vi "Add Injector.vi"(7 "Max Shots":T1(ring)=enum."1", 8 "error in (no error)":errorcluster, 9 "Stages":string[](array[string])=["Boost", "Battery", "Off"], 10 "Controls":T3[](array[typedef]) {"Data Type" format="%.0x"}, 11 "Item Ref":T2=18446744073709551615 format="%.0x") -> (0 "error out":errorcluster, 3 "Item Ref out":T2=18446744073709551615 format="%.0x")   [LabVIEW 2019, in "Fuel Injector Analysis Addon System Explorer.lvlib"]
uses:
  Fuel Injector Analysis Addon System Explorer.lvlib
  <vilib>/NI VeriStand/Custom Device API/Custom Device Item Ref.ctl
  Addon Shared/Types/Register.Info.ctl
  Addon Shared/Types/FPGA Data Types.ctl
  Support Libraries/Injection Capture IP/Types/Injection.Global.Settings.ctl
  Addon Shared/Constants.vi
  <vilib>/NI VeriStand/Custom Device API/Set Item Property (Variant).vi
  <vilib>/NI VeriStand/Custom Device Tools/Custom Device Utility Library/NI VeriStand - Search for Item by GUID.vi
  <vilib>/NI VeriStand/Custom Device Tools/Custom Device Utility Library/NI VeriStand - Search for All Items by GUID.vi
  Addon Shared/Fuel Injector Analysis Addon Shared.lvlib
  <vilib>/NI VeriStand/Custom Device API/Custom Device API.lvlib
  <vilib>/NI VeriStand/Custom Device Tools/Custom Device Utility Library/Custom Device Utility Library.lvlib
panel:
  in  "Tags":string
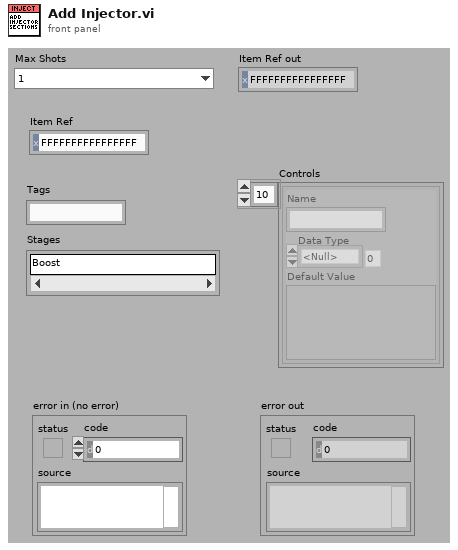
[diagram p1: front panel]
types:
  T1 = enum16{"0", "1", "2", "3", "4", "5", "6", "7", "8"}
  T2 = typedef "Custom Device API.lvlib/Custom Device Item Ref.ctl" = u64
  T3 = typedef "Fuel Injector Analysis Addon Shared.lvlib/Register.Info.ctl" = cluster{"Name":string, "Data Type":T4, "Default Value":variant}
  T4 = typedef "Fuel Injector Analysis Addon Shared.lvlib/FPGA Data Types.ctl" = enum8{"<Null>", "Injector.Core.Setting", "Injector.Global.Setting", "Injector.Mux.Setting", "Injector.Timing"}
  T5 = typedef "Injection.Global.Settings.ctl" = cluster{"Enable?":bool, "Initial Voltage Threshold":fxp<+/-,32,8>, "Event Dwell Limit":u16, "Voltage Gain":fxp<+/-,32,8>, "Current Gain":fxp<+/-,32,8>, "Filter Samples":u8, "Pretrigger Samples":u8, "Active Edge":bool}
  T6 = cluster{"Voltage Offset":fxp<+/-,32,8>, "Current Offset":fxp<+/-,32,8>}
  T7 = typedef "Custom Device API.lvlib/Custom Device Item Info.ctl" = cluster{"Name":string, "Is Channel":bool, "GUID":string, "Is Waveform":bool}
  T8 = typedef "Fuel Injector Analysis Addon Shared.lvlib/Main Settings.ctl" = cluster{"RIO Device Address":string, "Local bitfile path":path, "RT bitfile path":path, "Number of injectors":u16}
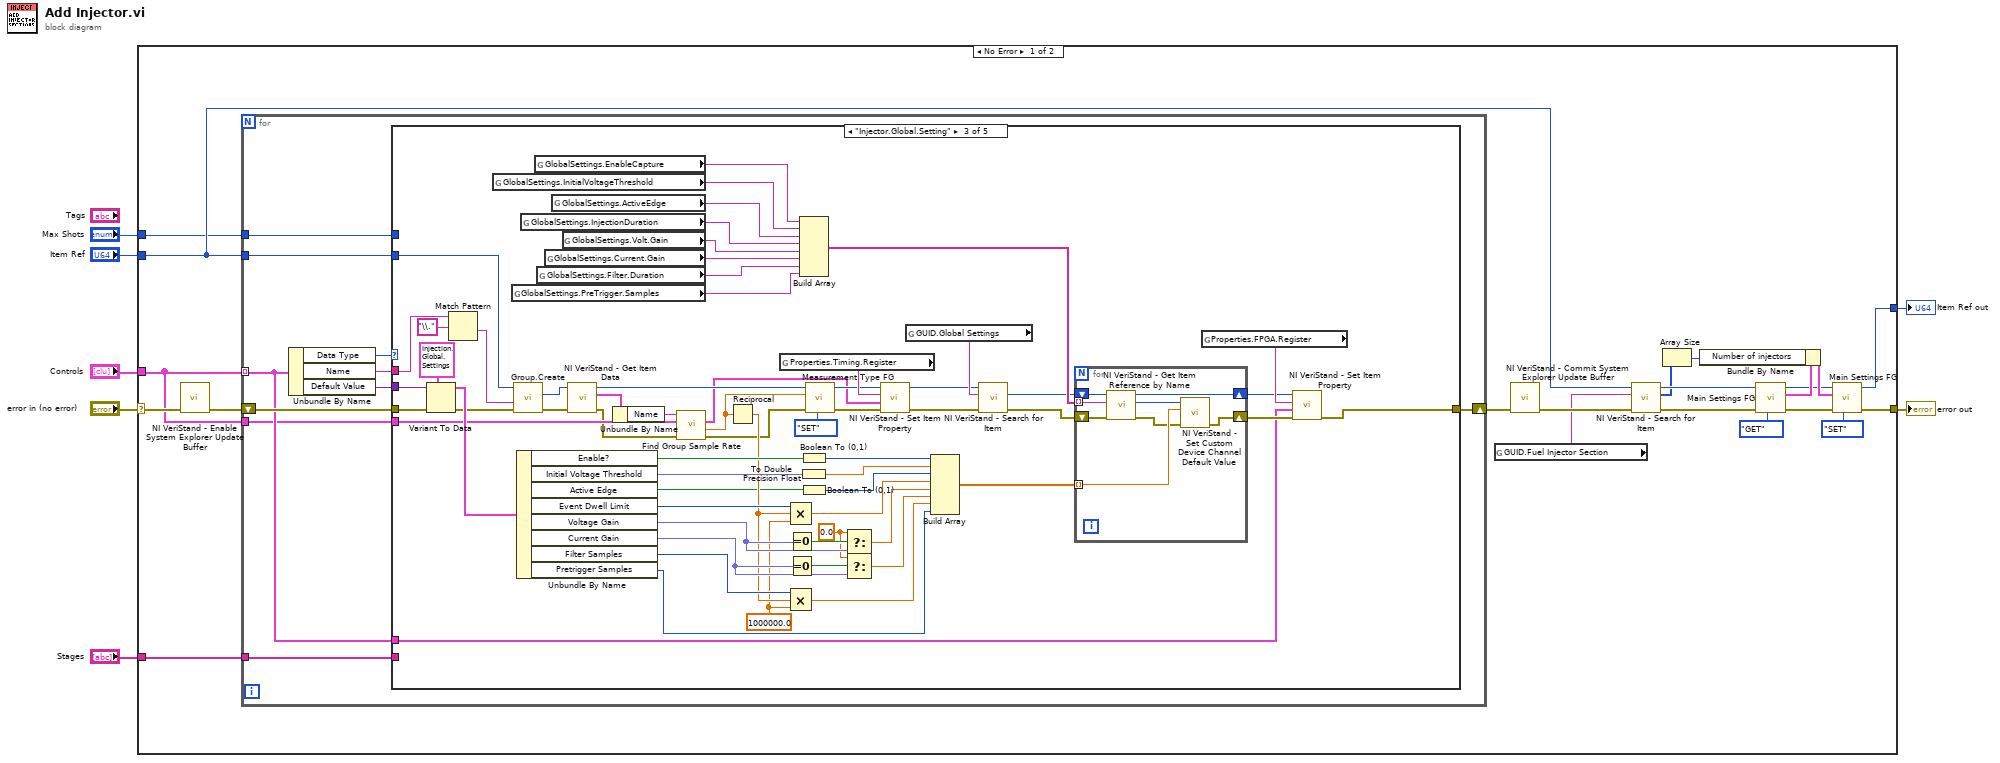
[diagram p0: block diagram]
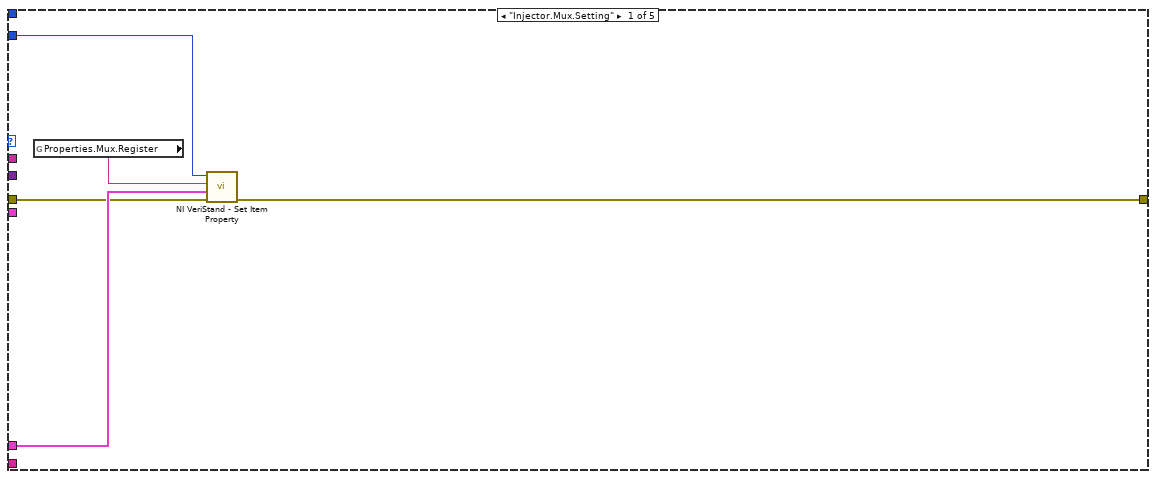
[diagram p2: hidden frame]
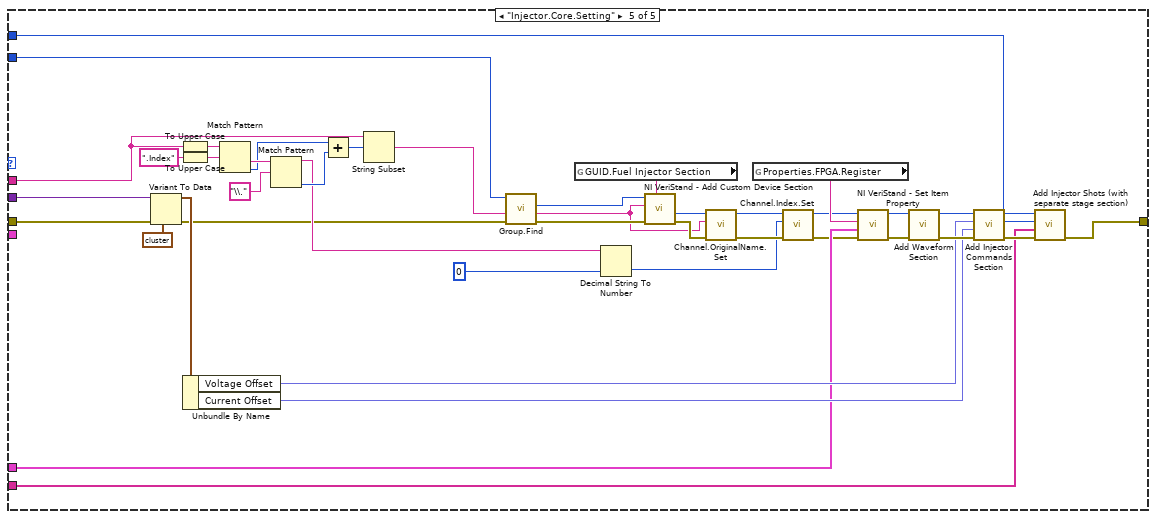
[diagram p5: hidden frame]
diagram:
  n1 = case shown="No Error" "error in (no error)" {
    selector: "error in (no error)" -> [w28 w160]
    tunnel: [w16 w160] -> w7
    tunnel: "Item Ref" -> [w21 w159]
    tunnel: "Controls" -> [w8 _]
    tunnel: [w15 w159] -> w3
    tunnel: "Stages" -> [w19 _]
    tunnel: "Max Shots" -> [w17 _]
    frame No Error {
      n2 = call <vilib>:"NI VeriStand - Enable System Explorer Update Buffer.vi"("error in (no error)"=w28) -> ("error out"=w20:errorcluster)  [unwired: 10 in]
      n3 = for {
        shift-right: [w37] -> w18
        shift-left: w20 -> [w38]
        tunnel: w8 -> [w35] mode=indexing
        tunnel: w19 -> [w32]
        tunnel: w17 -> [w31]
        tunnel: w21 -> [w30]
        tunnel: w8 -> [w29]
        n4 = Unbundle By Name(w35) -> ("Data Type"=w33:T4, "Name"=w34:string, "Default Value"=w36:variant)
        n5 = case shown="\"Injector.Global.Setting\"" w33 {
          tunnel: w38 -> [w40 w44 w62 w116 w152]
          tunnel: [w39 w44 w95 w116 w153] -> w37
          tunnel: w30 -> [w41 _ w63 _ w118]
          tunnel: w36 -> [_ _ w107 _ w151]
          tunnel: w35 -> [w42 _ w93 _ w143]
          tunnel: w34 -> [_ _ w67 _ w137]
          tunnel: w32 -> [_ _ _ _ w133]
          tunnel: w31 -> [_ _ _ _ w132]
          tunnel: w29 -> [_ _ w60 _ _]
          frame "Injector.Mux.Setting" {
            n6 = global read "Constants.vi" "Properties.Mux.Register"() -> (w43:string)
            n7 = call-poly <vilib>:"NI VeriStand - Set Item Property.vi"("error in (no error)"=w40, "Value"=w42, "Property Name"=w43, "Item Ref in"=w41) -> ("error out"=w39:errorcluster)  [unwired: 5 in, 2 out]
          }
          frame "Injector.Timing" {
            # "NOTE: Handled in the global settings and group creation"
          }
          frame "Injector.Global.Setting" {
            w71 = 1000000.0 ("value")
            w79 = 0.0 ("x*y")
            n8 = Variant To Data(error in=w62, type=T5 {"Enable?"=FALSE, "Initial Voltage Threshold"=0.0, "Event Dwell Limit"=0, "Voltage Gain"=0.0, "Current Gain"=1.0, "Filter Samples"=5, "Pretrigger Samples"=5, "Active Edge"=TRUE} ("InjectorAnalysis.Settings"), Variant=w107) -> (data=w106:T5, error out=w61:errorcluster)
            n9 = Match Pattern(string=w67, regular expression="\\.") -> (after substring=w68:string)  [unwired: 1 in, 3 out]
            n10 = global read "Constants.vi" "GlobalSettings.InitialVoltageThreshold"() -> (w77:string)
            n11 = global read "Constants.vi" "GlobalSettings.PreTrigger.Samples"() -> (w75:string)
            n12 = call "Group.Create.vi"("error in (no error)"=w61, "Name"=w68, "Parent"=w63) -> ("error out"=w59:errorcluster, "Child"=w57:T2)  [unwired: 6 in, 1 out]
            n13 = Unbundle By Name(w106) -> ("Enable?"=w100:bool, "Initial Voltage Threshold"=w101:fxp<+/-,32,8>, "Active Edge"=w65:bool, "Event Dwell Limit"=w98:u16, "Voltage Gain"=w92:fxp<+/-,32,8>, "Current Gain"=w91:fxp<+/-,32,8>, "Filter Samples"=w74:u8, "Pretrigger Samples"=w70:u8)
            n14 = global read "Constants.vi" "GlobalSettings.InjectionDuration"() -> (w88:string)
            n15 = global read "Constants.vi" "GlobalSettings.EnableCapture"() -> (w89:string)
            n16 = global read "Constants.vi" "GlobalSettings.Filter.Duration"() -> (w76:string)
            n17 = global read "Constants.vi" "GlobalSettings.Current.Gain"() -> (w86:string)
            n18 = global read "Constants.vi" "GlobalSettings.ActiveEdge"() -> (w66:string)
            n19 = global read "Constants.vi" "GlobalSettings.Volt.Gain"() -> (w87:string)
            n20 = call <vilib>:"NI VeriStand - Get Item Data.vi"("error in (no error)"=w59, "Item Ref in"=w57) -> ("error out"=w58:errorcluster, "Item Info"=w56:T7, "Item Ref out"=w50:T2)  [unwired: 6 in, 1 out]
            n21 = Unbundle By Name(w56) -> ("Name"=w55:string)
            n22 = call "Find Group Sample Rate.vi"("error in (no error)"=w58, "Controls"=w60, "group"=w55) -> ("error out"=w48:errorcluster, "Rate"=w46:dbl, "Register"=w45:T3)  [unwired: 6 in]
            n23 = Reciprocal(x=w46) -> (1/x=w73:dbl)
            n24 = global read "Constants.vi" "Properties.Timing.Register"() -> (w53:string)
            n25 = Equal To 0?(x=w92) -> (x = 0?=w83:bool)
            n26 = Equal To 0?(x=w91) -> (x = 0?=w80:bool)
            n27 = Compound Arithmetic op=MULTIPLY(w98, w73, w71) -> (w81:dbl)
            n28 = Compound Arithmetic op=MULTIPLY(w74, w73, w71) -> (w72:dbl)
            n29 = Build Array(w89, w77, w66, w88, w87, w86, w76, w75) -> (w103:string[])
            n30 = Boolean To (0,1)(Boolean=w100) -> (0, 1=w85:i16)
            n31 = To Double Precision Float(number=w101) -> (double precision float=w84:dbl)
            n32 = Boolean To (0,1)(Boolean=w65) -> (0, 1=w64:i16)
            n33 = call "Measurement Type FG.vi"("Action"=enum8{"GET", "SET"}."SET", "error in (no error)"=w48, "Sample rate (S/s)"=w46, "Item Ref"=w50) -> ("error out"=w52:errorcluster, "Item Ref out"=w51:T2)  [unwired: 5 in, 1 out]
            n34 = Select(t=w79, s=w83, f=w92) -> (s? t:f=w82:dbl)
            n35 = Select(t=w79, s=w80, f=w91) -> (s? t:f=w78:dbl)
            n36 = call-poly <vilib>:"NI VeriStand - Set Item Property.vi"("error in (no error)"=w52, "Value"=w45, "Property Name"=w53, "Item Ref in"=w51) -> ("error out"=w47:errorcluster, "Item Ref out"=w49:T2)  [unwired: 5 in, 1 out]
            n37 = global read "Constants.vi" "GUID.Global Settings"() -> (w104:string)
            n38 = Build Array(w85, w84, w64, w81, w82, w78, w72, w70) -> (w99:dbl[])
            n39 = call-poly <vilib>:"NI VeriStand - Search for Item.vi"("error in"=w47, "Item GUID"=w104, "Section Ref in"=w49) -> ("error out"=w102:errorcluster, "Item Ref"=w90:T2)  [unwired: 5 in, 2 out]
            n40 = for {
              tunnel: w103 -> [w112] mode=indexing
              shift-right: [w115] -> w96
              shift-left: w102 -> [w111]
              tunnel: w99 -> [w114] mode=indexing
              shift-right: [w109] -> w94
              shift-left: w90 -> [w113]
              n41 = call <vilib>:"NI VeriStand - Get Item Reference by Name.vi"("error in (no error)"=w111, "Item Name"=w112, "Parent Ref in"=w113) -> ("error out"=w110:errorcluster, "Item Ref"=w108:T2, "Parent Ref out"=w109:T2)  [unwired: 5 in, 1 out]
              n42 = call <vilib>:"NI VeriStand - Set Custom Device Channel Default Value.vi"("error in (no error)"=w110, "Default Value"=w114, "Channel Ref in"=w108) -> ("error out"=w115:errorcluster)  [unwired: 7 in, 1 out]
            }
            n43 = global read "Constants.vi" "Properties.FPGA.Register"() -> (w97:string)
            n44 = call-poly <vilib>:"NI VeriStand - Set Item Property.vi"("error in (no error)"=w96, "Value"=w93, "Property Name"=w97, "Item Ref in"=w94) -> ("error out"=w95:errorcluster)  [unwired: 5 in, 2 out]
          }
          frame "<Null>", Default {
          }
          frame "Injector.Core.Setting" {
            n45 = Variant To Data(error in=w152, type=T6 {"Voltage Offset"=0.0, "Current Offset"=0.0} ("Injector.Core.Settings Ch5"), Variant=w151) -> (data=w149:T6, error out=w122:errorcluster)
            n46 = To Upper Case(1:w137) -> (0:w141:string)
            n47 = To Upper Case(1:".Index" ("regular expression")) -> (0:w140:string)
            n48 = Unbundle By Name(w149) -> ("Voltage Offset"=w148:fxp<+/-,32,8>, "Current Offset"=w147:fxp<+/-,32,8>)
            n49 = Match Pattern(string=w141, regular expression=w140) -> (after substring=w139:string, offset past match=w136:i32)  [unwired: 1 in, 2 out]
            n50 = Match Pattern(string=w139, regular expression="\\.") -> (before substring=w129:string, offset past match=w135:i32)  [unwired: 1 in, 2 out]
            n51 = Add(x=w136, y=w135) -> (x+y=w134:i32)
            n52 = String Subset(string=w137, offset (0)=w134) -> (substring=w117:string)  [unwired: 1 in]
            n53 = call "Group.Find.vi"("error in (no error)"=w122, "Name"=w117, "Parent"=w118) -> ("error out"=w121:errorcluster, "Child Name"=w120:string, "Child"=w119:T2)  [unwired: 5 in, 1 out]
            n54 = global read "Constants.vi" "GUID.Fuel Injector Section"() -> (w156:string)
            n55 = Decimal String To Number(string=w129, default (0L)=u16 0 ("default (0 I32)")) -> (number=w123:u16)  [unwired: 1 in, 1 out]
            n56 = call <vilib>:"NI VeriStand - Add Custom Device Section.vi"("GUID (Default Section)"=w156, "error in (no error)"=w121, "Section Name"=w120, "Parent Ref in"=w119) -> ("error out"=w130:errorcluster, "Section Ptr"=w131:T2)  [unwired: 4 in, 2 out]
            n57 = call "Channel.OriginalName.Set.vi"("error in (no error)"=w130, "Constants.Channel Name"=w120, "Ref"=w131) -> ("error out"=w126:errorcluster, "Ref out"=w127:T2)  [unwired: 7 in]
            n58 = global read "Constants.vi" "Properties.FPGA.Register"() -> (w144:string)
            n59 = call "Channel.Index.Set.vi"("error in (no error)"=w126, "Constants.Index"=w123, "Ref"=w127) -> ("error out"=w124:errorcluster, "Ref out"=w125:T2)  [unwired: 7 in]
            n60 = call-poly <vilib>:"NI VeriStand - Set Item Property.vi"("error in (no error)"=w124, "Value"=w143, "Property Name"=w144, "Item Ref in"=w125) -> ("error out"=w146:errorcluster, "Item Ref out"=w145:T2)  [unwired: 5 in, 1 out]
            n61 = call "Add Waveform Section.vi"("error in (no error)"=w146, "Section Ptr"=w145) -> ("error out"=w158:errorcluster, "Injector Section ptr"=w157:T2)  [unwired: 8 in]
            n62 = call "Add Injector Commands Section.vi"("error in (no error)"=w158, "Default Current Offset"=w147, "Default Volt Offset"=w148, "Injector Section ptr"=w157) -> ("error out"=w154:errorcluster, "Parent Ref out"=w155:T2)  [unwired: 6 in]
            n63 = call "Add Injector Shots (with separate stage section).vi"("error in (no error)"=w154, "Stage Names"=w133, "# shots to add"=w132, "Injector Section Ref in"=w155) -> ("error out"=w153:errorcluster)  [unwired: 7 in]
          }
        }
      }
      n64 = global read "Constants.vi" "GUID.Fuel Injector Section"() -> (w11:string)
      n65 = call <vilib>:"NI VeriStand - Commit System Explorer Update Buffer.vi"("error in (no error)"=w18) -> ("error out"=w14:errorcluster)  [unwired: 10 in]
      n66 = call-poly <vilib>:"NI VeriStand - Search for Item.vi"("error in"=w14, "Item GUID"=w11, "Section Ref in"=w21) -> ("error out"=w13:errorcluster, "Item Refs"=w10:T2[], "Section Ref out"=w12:T2)  [unwired: 5 in, 1 out]
      n67 = Array Size(array=w10) -> (size(s)=w9:i32)
      n68 = call "Main Settings FG.vi"("Action"=enum8{"GET", "SET"}."GET", "error in (no error)"=w13, "Item Ref"=w12) -> ("error out"=w27:errorcluster, "Main Settings out"=w26:T8, "Item Ref out"=w23:T2)  [unwired: 6 in]
      n69 = Bundle By Name(cluster=w26, "Number of injectors"=w9) -> (w25:T8)
      n70 = call "Main Settings FG.vi"("Action"=enum8{"GET", "SET"}."SET", "error in (no error)"=w27, "Main Settings"=w25, "Item Ref"=w23) -> ("error out"=w16:errorcluster, "Item Ref out"=w15:T2)  [unwired: 5 in, 1 out]
    }
    frame Error {
    }
  }
  "error out" <- w7
  "Item Ref out" <- w3
